vi "Einheiten in Tabellenspalten.vi"(8 "error in (no error)":errorcluster caption="Fehler (Eingang, kein Fehler)", 9 "Spalten Titel mit Einheiten in":string[](array[string])=["Setpoint\n---", "Raw Value\n[%]", "Linearized\n[ppm]", "abs.Error\n[ppm[ppm[ppm[ppm[ppm]", "rel.Error\n% from Setpoint", "Deviation\n[ppm[ppm[ppm[ppm[ppm]", "Temp. Gascell\nin °C", "Pressure Gascell\nin atm", ""], 10 "Einheit":string, 11 "Tabelle (Eingang)":refnum<vi>) -> (0 "error out":errorcluster caption="Fehler (Ausgang)", 2 "Einheit out":string, 3 "Spalten Titel mit Einheiten out":string[](array[string]))   [LabVIEW 2020, in "Linearisierung v2.lvlib"]
uses:
  Linearisierung v2.lvlib
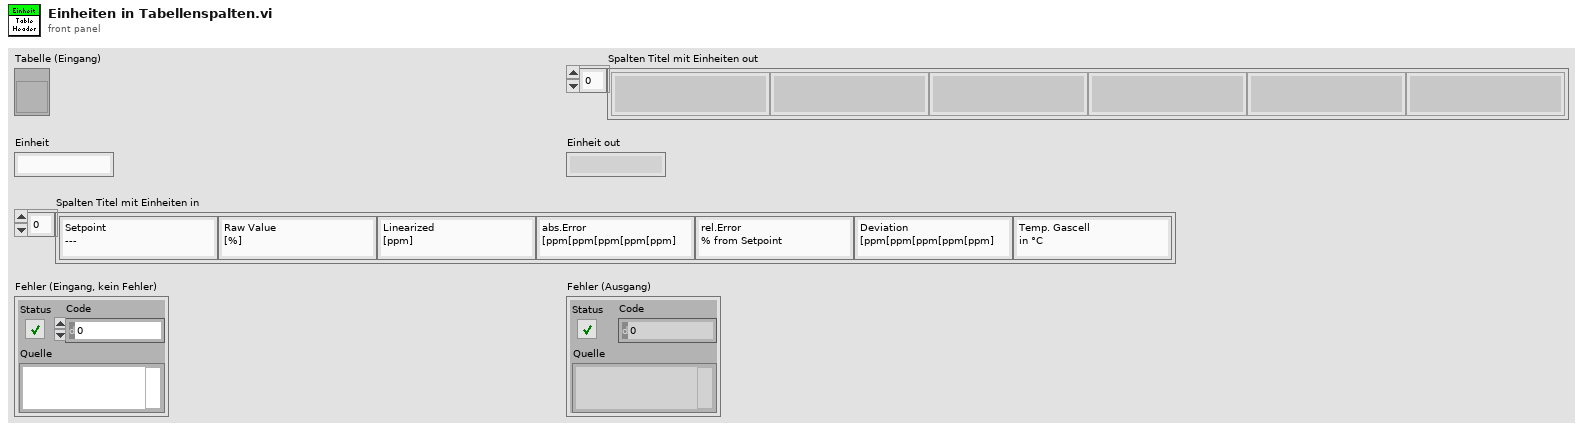
[diagram p1: front panel]
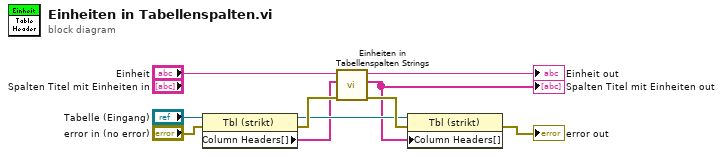
[diagram p0: block diagram]
diagram:
  n1 = property on="Eigenschaftsknoten" class="Tbl (strikt)"(reference="Tabelle (Eingang)", error in="error in (no error)") -> (reference out=w5:refnum<vi>, error out=w8:errorcluster, "Column Headers[]"=w1:string[])
  n2 = call "Einheiten in Tabellenspalten Strings.vi"("Fehler (Eingang, kein Fehler)"=w8, "Spalten Titel mit Einheiten in"=w1, "Einheit in"="Einheit") -> ("Fehler (Ausgang)"=w7:errorcluster, "Spalten Titel mit Einheiten out"=w4:string[], "Einheit out"=→"Einheit out":string)  [unwired: 6 in]
  "Spalten Titel mit Einheiten out" <- w4
  n3 = property on="Eigenschaftsknoten" class="Tbl (strikt)"(reference=w5, error in=w7, "Column Headers[]"=w4) -> (error out=→"error out":errorcluster)  [unwired: 1 out]
